vi "SPIM_Video2.vi"() -> ()   [LabVIEW 2012]
panel:
  in  "Convert":bool
  out "Progress":u8(slide)=99 scale=0.0..100.0
  in  "Destination Path 2":path=path "H:/P13_.AVI"
  out "Total Frames":i32=200
  out "Image":T1(plugin-control)
  out "error out":errorcluster
  in  "Source Path":path=path "D:/BackUp Data/zb-20x-new_S16_head_700mV_GCamp.ps"
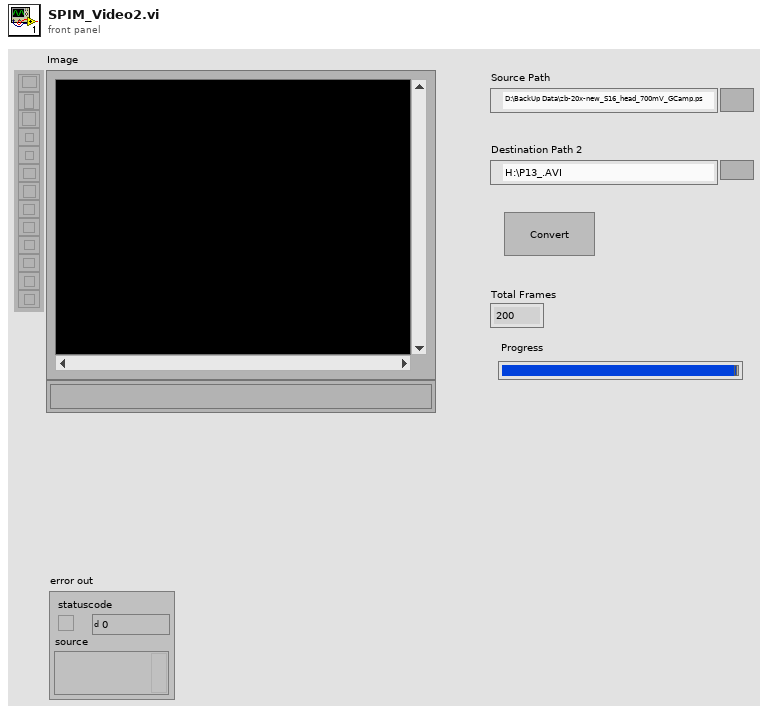
[diagram p1: front panel]
types:
  T1 = typedef "IMAQ Image.ctl" = refnum<image>
  T2 = typedef "Image Type" = u32
  T3 = typedef "AviRefnum.ctl" = refnum<k1>
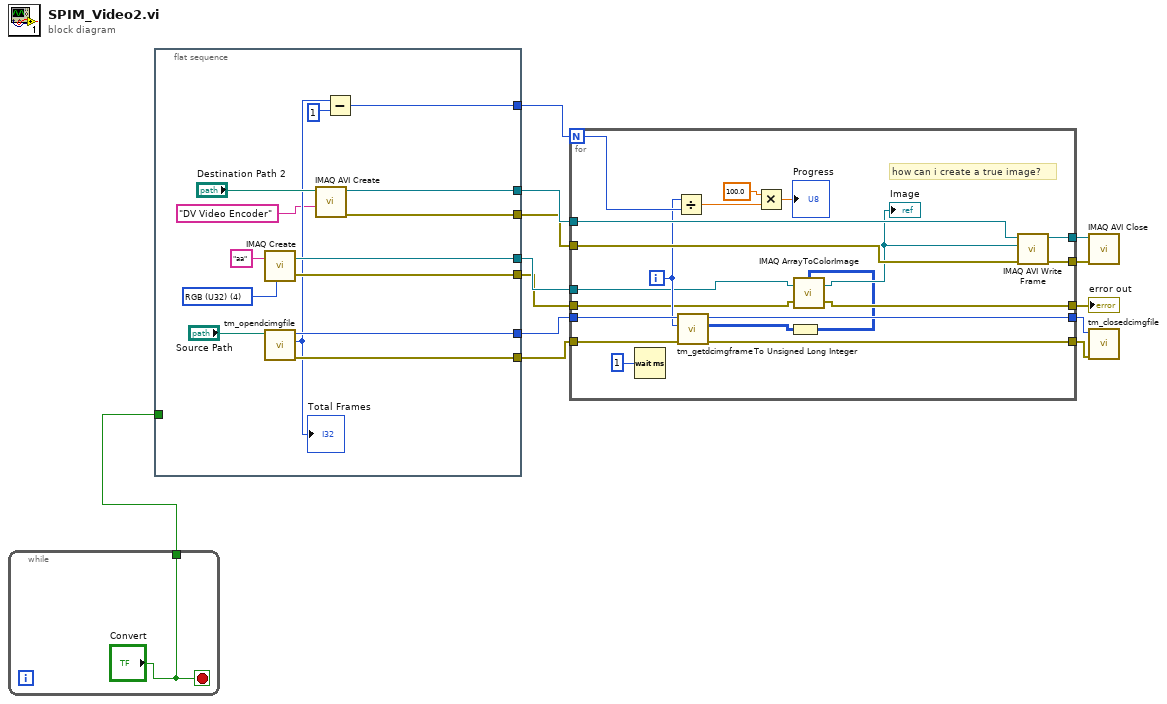
[diagram p0: block diagram]
diagram:
  n1 = while {
    tunnel: ["Convert"] -> w1
    stop <- "Convert" stop-if-true
  }
  n2 = flat-sequence {
    tunnel: [w26] -> w13
    tunnel: [w25] -> w11
    tunnel: [w23] -> w10
    tunnel: [w22] -> w9
    tunnel: [w20] -> w6
    tunnel: [w19] -> w5
    tunnel: [w16] -> w2
    tunnel: w1 -> [_]
    frame #0 {
      w24 = T2 4 items=["Grayscale (U8)", "Grayscale (I16)", "Grayscale (SGL)", "Complex (CSG)", "RGB (U32)", "HSL (U32)", "RGB (U64)"] ("Image Type")
      n3 = call "IMAQ Create"("Image Name"="aa", "Image Type"=w24) -> ("New Image"=w26:T1, "error out"=w25:errorcluster)  [unwired: 3 in]
      n4 = call <userlib>:"tm_opendcimgfile.vi"("Path"="Source Path") -> ("error out"=w22:errorcluster, "Total Frames"=w18:i32, "File Handle"=w23:u32)  [unwired: 8 in]
      "Total Frames" <- w18
      n5 = call "IMAQ AVI Create"("Compression Filter"="DV Video Encoder", "AVI Path"="Destination Path 2") -> ("error out"=w19:errorcluster, "Avi Refnum"=w20:T3)  [unwired: 8 in]
      n6 = Subtract(x=w18, y=1) -> (x-y=w16:i32)
    }
  }
  n7 = for {
    N: w2 -> [w39]
    tunnel: w13 -> [w34]
    tunnel: [w32] -> w12
    tunnel: w11 -> [w31]
    tunnel: w10 -> [w48]
    tunnel: w9 -> [w47]
    tunnel: [w45] -> w8
    tunnel: [w44] -> w7
    tunnel: w6 -> [w43]
    tunnel: w5 -> [w42]
    tunnel: [w41] -> w4
    tunnel: [w40] -> w3
    i -> [w38]
    # "how can i create a true image?"
    n8 = Wait (ms)(milliseconds to wait=u32 1) -> ()  [unwired: 1 out]
    n9 = Divide(x=w38, y=w39) -> (x/y=w36:dbl)
    n10 = call <userlib>:"tm_getdcimgframe.vi"("error in (no error)"=w47, "Frame Index"=w38, "File Handle in"=w48) -> ("error out"=w44:errorcluster, "Data"=w30:u16[][], "File Handle out"=w45:u32)  [unwired: 5 in, 1 out]
    n11 = Multiply(x=100.0, y=w36) -> (x*y=→"Progress":dbl)
    n12 = To Unsigned Long Integer(number=w30) -> (unsigned 32bit integer=w29:u32[][])
    n13 = call "IMAQ ArrayToColorImage"("Image Pixels (U32)"=w29, "Image"=w34, "error in (no error)"=w31) -> ("Image Out"=w33:T1, "error out"=w32:errorcluster)  [unwired: 2 in]
    "Image" <- w33
    n14 = call "IMAQ AVI Write Frame"("error in (no error)"=w42, "Image"=w33, "Avi Refnum"=w43) -> ("error out"=w40:errorcluster, "Avi Refnum (duplicate)"=w41:T3)  [unwired: 7 in]
  }
  "error out" <- w12
  n15 = call "IMAQ AVI Close"("error in (no error)"=w3, "Avi Refnum"=w4) -> ()  [unwired: 9 in, 1 out]
  n16 = call <userlib>:"tm_closedcimgfile.vi"("error in (no error)"=w7, "File Handle"=w8) -> ()  [unwired: 9 in, 1 out]
